vi "BigEndianToLittleEndian_IP.vi"(11 "IP String":string) -> (3 "IP Network Order":u32)   [LabVIEW 2017, in "BonTechDetector.lvlib"]
uses:
  BonTechDetector.lvlib
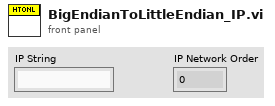
[diagram p1: front panel]
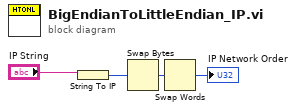
[diagram p0: block diagram]
diagram:
  n1 = String To IP(1:"IP String") -> (0:w3:u32)
  n2 = Swap Bytes(anything=w3) -> (byte swapped=w4:u32)
  n3 = Swap Words(1:w4) -> (0:→"IP Network Order":u32)
